vi "Read FeedbackData.vi"(8 "error in (no error)":errorcluster, 11 "RobotFeedback in":refnum<class "RobotFeedback.lvclass">) -> (0 "error out":errorcluster, 2 "FeedbackData":T1, 3 "RobotFeedback out":refnum<class "RobotFeedback.lvclass">)   [LabVIEW 2023, in "RobotFeedback.lvclass"]
uses:
  RobotFeedback.lvclass
  Communication_class/feedbackData.ctl
  RobotFeedback.lvclass/RobotFeedback.ctl
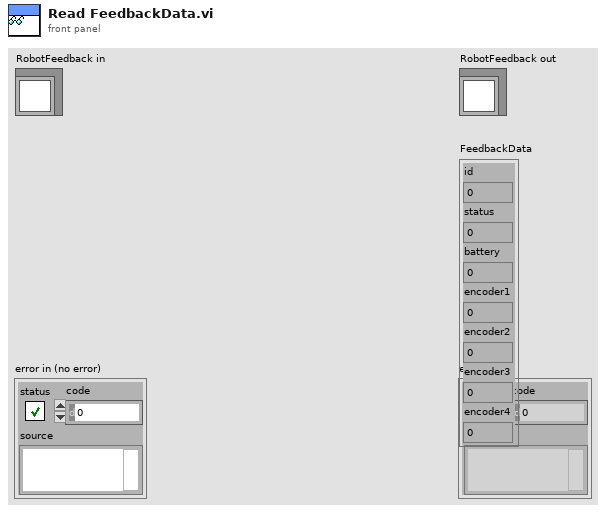
[diagram p1: front panel]
types:
  T1 = typedef "feedbackData.ctl" = cluster{"id":u32, "status":u32, "battery":sgl, "encoder1":sgl, "encoder2":sgl, "encoder3":sgl, "encoder4":sgl}
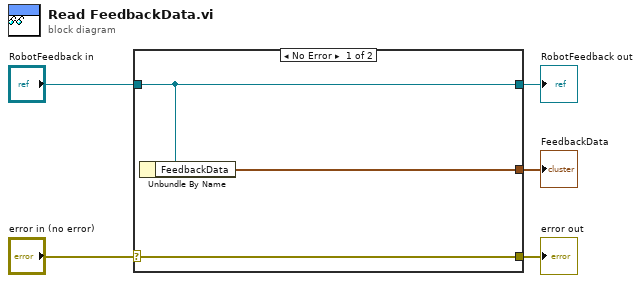
[diagram p0: block diagram]
diagram:
  n1 = case shown="No Error" "error in (no error)" {
    selector: "error in (no error)" -> [w8 w9]
    tunnel: [w8 w9] -> w4
    tunnel: [w7 w10] -> w2
    tunnel: "RobotFeedback in" -> [w7 w10]
    tunnel: [w6 _] -> w1
    frame No Error {
      n2 = Unbundle By Name(w7) -> ("FeedbackData"=w6:T1)
    }
    frame Error {
    }
  }
  "error out" <- w4
  "RobotFeedback out" <- w2
  "FeedbackData" <- w1
